vi "uTTA_SetSystemTime.vi"(8 "error in":errorcluster, 9 "Parameter":enum16{"Date", "Time", "Date+Time"}(ring), 10 "Time Stamp":timestamp format="%<%x %X>T", 11 "VISA Refnum in":refnum<visa-resource-name>) -> (0 "error out":errorcluster, 3 "VISA Refnum out":refnum<visa-resource-name>)   [LabVIEW 2021]
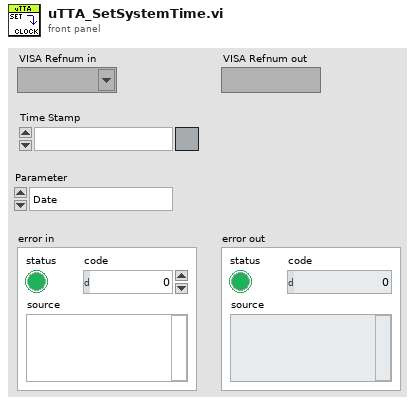
[diagram p1: front panel]
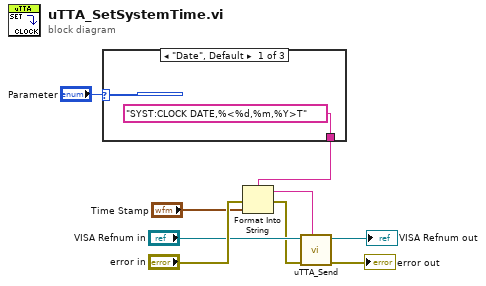
[diagram p0: block diagram]
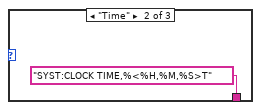
[diagram p2: hidden frame]
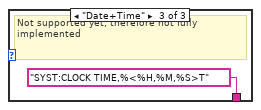
[diagram p3: hidden frame]
diagram:
  n1 = case shown="\"Date\", Default" "Parameter" {
    tunnel: ["SYST:CLOCK DATE,%<%d,%m,%Y>T" ("format string") "SYST:CLOCK TIME,%<%H,%M,%S>T" ("format string") "SYST:CLOCK TIME,%<%H,%M,%S>T" ("format string")] -> w8
    frame "Date", Default {
    }
    frame "Time" {
    }
    frame "Date+Time" {
      # "Not supported yet, therefore not fully implemented"
    }
  }
  n2 = Format Into String(format string=w8, error in="error in", "Time Stamp") -> (resulting string=w1:string, error out=w4:errorcluster)  [unwired: 1 in]
  n3 = call "uTTA_Send.vi"("Send String"=w1, "error in (no error)"=w4, "VISA Refnum in"="VISA Refnum in") -> ("error out"=→"error out":errorcluster, "VISA Refnum out"=→"VISA Refnum out":refnum<visa-resource-name>)  [unwired: 7 in]
